vi "Run_Test.vi"(8 "error in (no error)":errorcluster caption="entrée d'erreur (pas d'erreur)", 11 "Test (Default) en entrée":refnum<class "Sequencer (Default).lvclass">) -> (0 "error out":errorcluster caption="sortie d'erreur", 3 "Test (Default) en sortie":refnum<class "Sequencer (Default).lvclass">)   [LabVIEW 2020, in "Library Core.lvlib" / "Sequencer (Default).lvclass"]
uses:
  Sequencer (Default).lvclass
  Sequencer (Default).lvclass/Sequencer (Default).ctl
  0f25eb4b-c598-48e2-9928-b161e7f39afd.vi
  Variable Test.vi
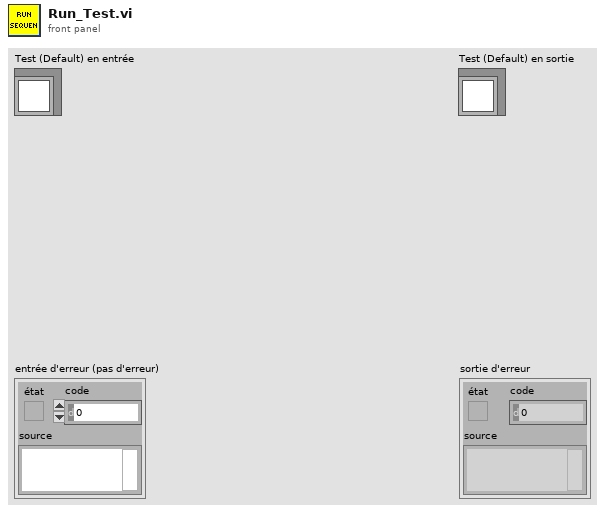
[diagram p1: front panel]
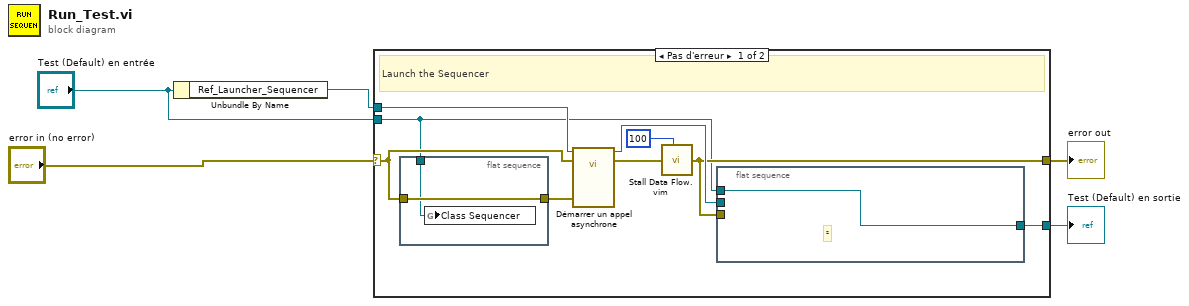
[diagram p0: block diagram]
diagram:
  n1 = Unbundle By Name("Test (Default) en entrée") -> ("Ref_Launcher_Sequencer"=w5:refnum<vi>)
  n2 = case shown="Pas d'erreur" "error in (no error)" {
    selector: "error in (no error)" -> [w8 w19]
    tunnel: [w9 w19] -> w2
    tunnel: [w14 w18] -> w1
    tunnel: "Test (Default) en entrée" -> [w6 w18]
    tunnel: w5 -> [w12 _]
    frame No Error {
      # "Launch the Sequencer"
      n3 = flat-sequence {
        tunnel: [w16] -> w7
        tunnel: w8 -> [w16]
        tunnel: w6 -> [w15]
        frame #0 {
          n4 = global write "Variable Test.vi" "Class Sequencer"(w15) -> ()
        }
      }
      n5 = call-by-ref "Démarrer un appel asynchrone"(reference=w12, error in=w8, 8:"error in (no error)"=w7) -> (reference out=w10:refnum<vi>, error out=w13:errorcluster)  [unwired: 7 in, 4 out]
      n6 = call "Stall Data Flow.vim"("value in"=w13, "milliseconds to wait"=u32 100) -> ("value out"=w9:errorcluster)  [unwired: 1 out]
      n7 = flat-sequence {
        tunnel: [w17] -> w14
        tunnel: w6 -> [w17]
        tunnel: w10 -> [_]
        tunnel: w9 -> [_]
        frame #0 {
          # "²"
        }
      }
    }
    frame Error {
    }
  }
  "error out" <- w2
  "Test (Default) en sortie" <- w1
